vi "LVFunction_Calculer la taille de la representation graphique d'un HASO.vi"(1 "Plot Area:Size 2":cluster{"Width":u32, "Height":u32}, 2 "Size":T1) -> (0 "Plot Area:Size":cluster{"Width":u32, "Height":u32})   [LabVIEW 2020]
uses:
  Point2D.ctl
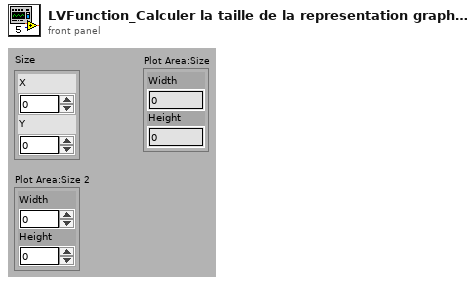
[diagram p1: front panel]
types:
  T1 = typedef "Point2D.ctl" = cluster{"X":u32, "Y":u32}
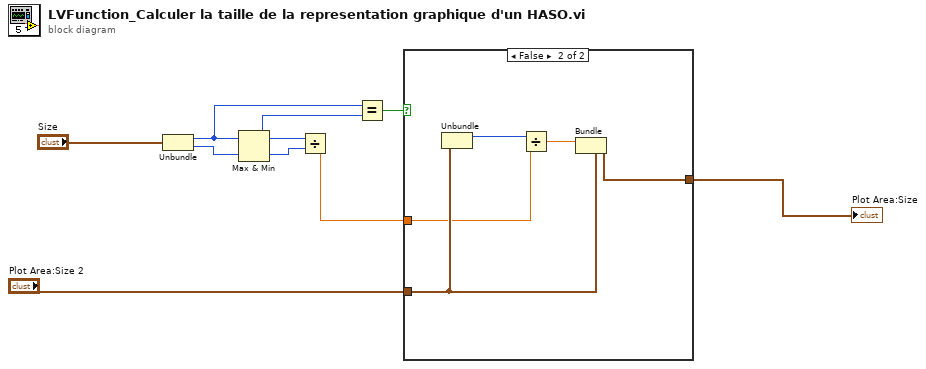
[diagram p0: block diagram]
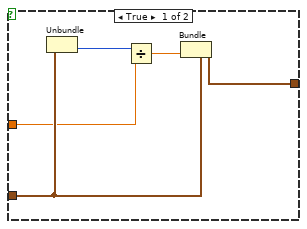
[diagram p2: hidden frame]
diagram:
  n1 = Unbundle("Size") -> ("X"=w2:u32, "Y"=w1:u32)
  n2 = Max & Min(x=w2, y=w1) -> (max(x,y)=w3:u32, min(x,y)=w4:u32)
  n3 = Divide(x=w3, y=w4) -> (x/y=w6:dbl)
  n4 = Equal?(x=w2, y=w3) -> (x = y?=w5:bool)
  n5 = case shown="False" w5 {
    tunnel: "Plot Area:Size 2" -> [w14 w19]
    tunnel: w6 -> [w13 w17]
    tunnel: [w11 w16] -> w8
    frame True {
      n6 = Unbundle(w14) -> ("Height"=w10:u32)  [unwired: 1 out]
      n7 = Divide(x=w10, y=w13) -> (x/y=w12:dbl)
      n8 = Bundle(cluster=w14, "Height"=w12) -> (w11:cluster{"Width":u32, "Height":u32})  [unwired: 1 in]
    }
    frame False {
      n9 = Unbundle(w19) -> ("Width"=w18:u32)  [unwired: 1 out]
      n10 = Divide(x=w18, y=w17) -> (x/y=w15:dbl)
      n11 = Bundle(cluster=w19, "Width"=w15) -> (w16:cluster{"Width":u32, "Height":u32})  [unwired: 1 in]
    }
  }
  "Plot Area:Size" <- w8
